vi "readConfig.vi"(8 "error in (no error)":errorcluster, 9 "config":string, 10 "deviceName":string, 11 "Ao8FileReader in":refnum<class "Ao8FileReader.lvclass">) -> (0 "error out":errorcluster, 3 "Ao8FileReader out":refnum<class "Ao8FileReader.lvclass">)   [LabVIEW 2011, in "Tools.lvlib" / "Filing.lvlib" / "Ao8FileReader.lvclass"]
uses:
  Ao8FileReader.lvclass
  Hal/Channels/VoltOutput/AnalogOutput.lvclass
  Ao8FileReader.lvclass/Ao8FileReader.ctl
  FileReader.lvclass
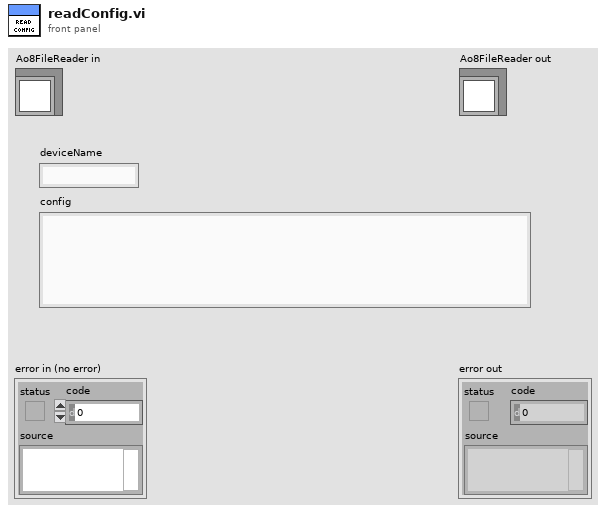
[diagram p1: front panel]
types:
  T1 = cluster{"Clock source":string, "Clock rate":dbl, "Start trigger line":string, "Sample Rate":dbl, "Sample No.":dbl}
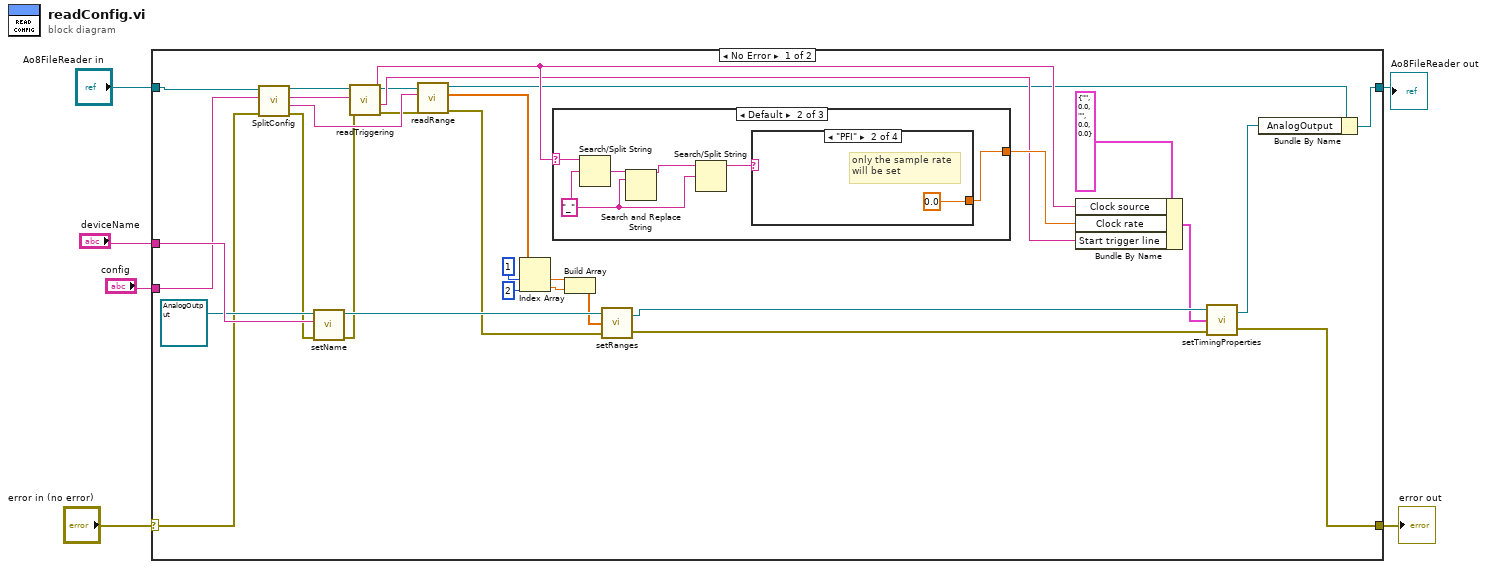
[diagram p0: block diagram]
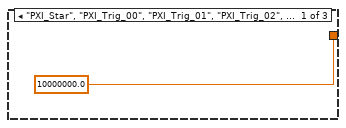
[diagram p2: hidden frame]
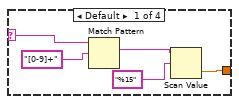
[diagram p3: hidden frame]
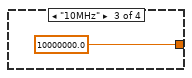
[diagram p4: hidden frame]
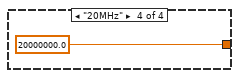
[diagram p5: hidden frame]
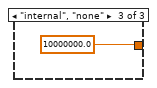
[diagram p6: hidden frame]
diagram:
  n1 = case shown="No Error" "error in (no error)" {
    selector: "error in (no error)" -> [w21 w54]
    tunnel: "Ao8FileReader in" -> [w22 w55]
    tunnel: [w28 w55] -> w5
    tunnel: [w7 w54] -> w3
    tunnel: "config" -> [w19 _]
    tunnel: "deviceName" -> [w35 _]
    frame No Error {
      n2 = call "SplitConfig.vi"("error in (no error)"=w21, "Config"=w19, "FileReader in"=w22) -> ("error out"=w20:errorcluster, "Range"=w13:string, "triggering"=w17:string, "FileReader out"=w18:refnum<class "Ao8FileReader.lvclass">)  [unwired: 4 in, 1 out]
      n3 = call "setName.vi"("error in (no error)"=w20, "name"=w35, "AnalogOutput.lvclass in"=refnum<class "AnalogOutput.lvclass"> refnum ("Hardware:Channels.lvlib:AnalogOutput.lvclass")) -> ("error out"=w11:errorcluster, "AnalogOutput.lvclass out"=w33:refnum<class "AnalogOutput.lvclass">)  [unwired: 7 in]
      n4 = call-dynamic "readTriggering.vi"("error in (no error)"=w11, "triggering"=w17, "FileReader in"=w18) -> ("error out"=w12:errorcluster, "start trigger line"=w15:string, "clock source"=w16:string, "FileReader out"=w14:refnum<class "Ao8FileReader.lvclass">)  [unwired: 5 in]
      n5 = call-dynamic "readRange.vi"("error in (no error)"=w12, "range"=w13, "FileReader in"=w14) -> ("error out"=w10:errorcluster, "range"=w9:dbl[], "FileReader out"=w8:refnum<class "Ao8FileReader.lvclass">)  [unwired: 6 in]
      n6 = Index Array(array=w9, index #1=1 ("index"), index #2=2 ("index")) -> (element #1=w24:dbl, element #2=w25:dbl)
      n7 = case shown="Default" w16 {
        selector: w16 -> [_ w42 _]
        tunnel: [10000000.0 w44 10000000.0] -> w31
        frame "PXI_Star", "PXI_Trig_00", "PXI_Trig_01", "PXI_Trig_02", "PXI_Trig_03", "PXI_Trig_04", "PXI_Trig_05", "PXI_Trig_06", "PXI_Trig_07" {
        }
        frame Default {
          w40 = "_"
          n8 = Search/Split String(string=w42, search string/char (-)=w40) -> (match + rest of string=w41:string)  [unwired: 1 in, 2 out]
          n9 = Search and Replace String(input string=w41, search string=w40) -> (result string=w39:string)  [unwired: 6 in, 3 out]
          n10 = Search/Split String(string=w39, search string/char (-)=w40) -> (substring before match=w43:string)  [unwired: 1 in, 2 out]
          n11 = case shown="\"PFI\"" w43 {
            selector: w43 -> [w49 _ _ _]
            tunnel: [w47 0.0 10000000.0 20000000.0] -> w44
            frame Default {
              n12 = Match Pattern(string=w49, regular expression="[0-9]+") -> (match substring=w46:string)  [unwired: 1 in, 3 out]
              n13 = Scan Value(string=w46, format string="%15") -> (value=w47:dbl)  [unwired: 1 in, 1 out]
            }
            frame "PFI" {
              # "only the sample rate\nwill be set"
            }
            frame "10MHz" {
            }
            frame "20MHz" {
            }
          }
        }
        frame "internal", "none" {
        }
      }
      n14 = Build Array(w24, w25) -> (w23:dbl[])
      n15 = call "setRanges.vi"("error in (no error)"=w10, "Ranges"=w23, "AnalogOutput.lvclass in"=w33) -> ("error out"=w36:errorcluster, "AnalogOutput.lvclass out"=w37:refnum<class "AnalogOutput.lvclass">)
      n16 = Bundle By Name(cluster=T1 {"Clock source"="", "Clock rate"=0.0, "Start trigger line"="", "Sample Rate"=0.0, "Sample No."=0.0} ("Timing"), "Clock source"=w16, "Clock rate"=w31, "Start trigger line"=w15) -> (w30:T1)
      n17 = call "setTimingProperties.vi"("error in (no error)"=w36, "Timing"=w30, "AnalogOutput.lvclass in"=w37) -> ("error out"=w7:errorcluster, "AnalogOutput.lvclass out"=w29:refnum<class "AnalogOutput.lvclass">)
      n18 = Bundle By Name(cluster=w8, "AnalogOutput"=w29) -> (w28:refnum<class "Ao8FileReader.lvclass">)
    }
    frame Error {
    }
  }
  "error out" <- w3
  "Ao8FileReader out" <- w5
